vi "Lab04_Correct.vi"() -> ()   [LabVIEW 2022 SP3]
uses:
  <vilib>/measure/NI_MABase.lvlib
panel:
  out "Waveform Graph 2":dbl[](graph)
  in  "Number of Waves":i32 min=0 max=250
  out "Waveform Graph":waveform(dbl)[](graph)
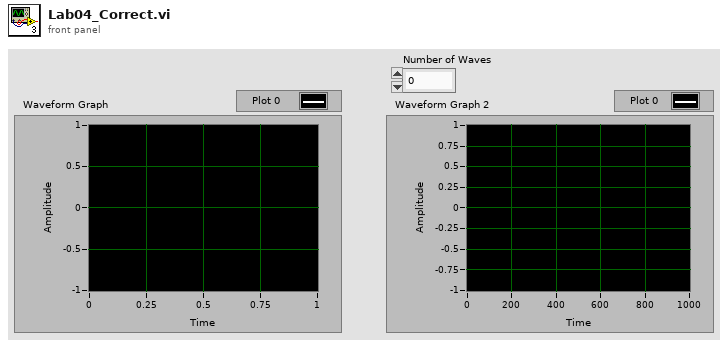
[diagram p1: front panel]
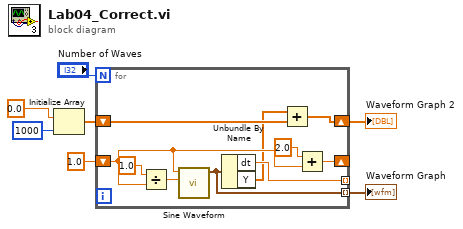
[diagram p0: block diagram]
diagram:
  n1 = Initialize Array(0.0 ("element"), 1000 ("dimension size")) -> (w3:dbl[])
  n2 = for {
    N: "Number of Waves" -> [_]
    shift-right: [w15] -> _
    shift-left: 1.0 -> [w13]
    tunnel: [w14] -> w2 mode=indexing
    tunnel: [w11] -> _ mode=indexing
    shift-right: [w8] -> w1
    shift-left: w3 -> [w10]
    n3 = Divide(x=1.0, y=w13) -> (x/y=w16:dbl)
    n4 = call <vilib>:"Sine Waveform.vi"("amplitude"=w16, "frequency"=w13) -> ("signal out"=w14:waveform(dbl))  [unwired: 8 in, 1 out]
    n5 = Unbundle By Name(w14) -> ("dt"=w11:dbl, "Y"=w9:dbl[])
    n6 = Add(x=w9, y=w10) -> (x+y=w8:dbl[])
    n7 = Add(x=2.0, y=w13) -> (x+y=w15:dbl)
  }
  "Waveform Graph" <- w2
  "Waveform Graph 2" <- w1
